vi "GV_DrawLiveBox.vi"(8 "error in (no error)":errorcluster, 11 "Gviewer in":refnum<class "Gviewer.lvclass">) -> (0 "error out":errorcluster, 3 "Gviewer out":refnum<class "Gviewer.lvclass">)   [LabVIEW 2020, in "Gviewer.lvclass"]
doc: "Position Live box on toolbar and update value from attributes"
uses:
  Gviewer.lvclass
  <vilib>/Utility/miscctls.llb/LVPositionTypeDef.ctl
  Gviewer.lvclass/Gviewer.ctl
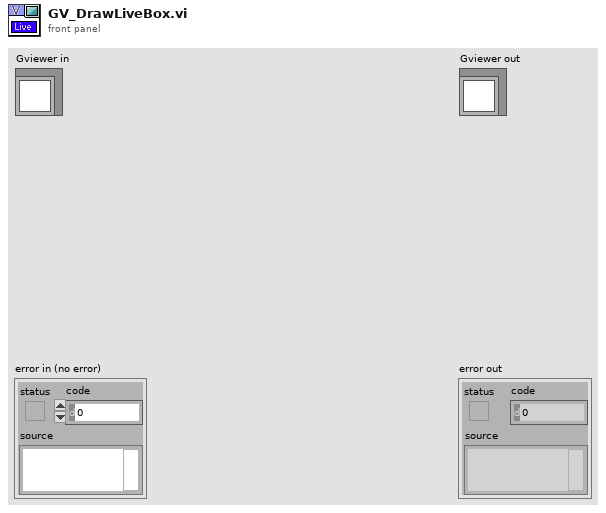
[diagram p1: front panel]
types:
  T1 = typedef "LVPositionTypeDef.ctl" = cluster{"Left":i32, "Top":i32}
  T2 = typedef "Gviewer.lvclass/Typedef_Live.ctl" = enum16{"Live View", "Freeze"}
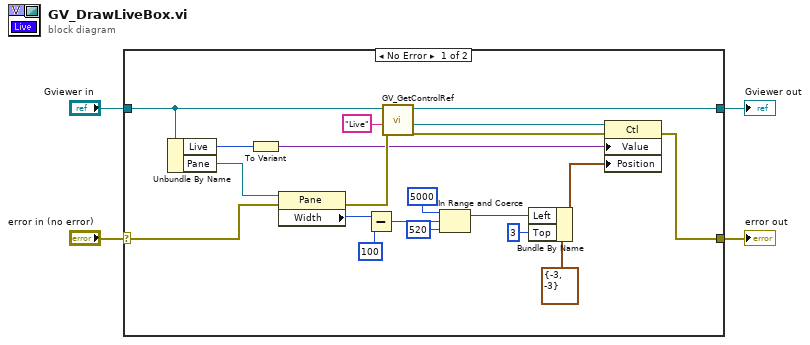
[diagram p0: block diagram]
diagram:
  n1 = case shown="No Error" "error in (no error)" {
    selector: "error in (no error)" -> [w17 w26]
    tunnel: [w16 w26] -> w3
    tunnel: [w18 w25] -> w1
    tunnel: "Gviewer in" -> [w19 w25]
    frame No Error {
      n2 = Unbundle By Name(w19) -> ("Live"=w10:T2, "Pane"=w20:refnum<vi>)
      n3 = To Variant(anything=w10) -> (Variant=w9:variant)
      n4 = property class="Pane"(reference=w20, error in=w17) -> (error out=w21:errorcluster, "Width"=w14:u32)  [unwired: 1 out]
      n5 = Subtract(x=w14, y=u32 100) -> (x-y=w8:u32)
      n6 = call "GV_GetControlRef.vi"("error in (no error)"=w21, "CNT name"="Live", "Gviewer in"=w19) -> ("error out"=w22:errorcluster, "Reference"=w23:refnum<vi>, "Gviewer out"=w18:refnum<class "Gviewer.lvclass">)  [unwired: 6 in]
      n7 = In Range and Coerce(upper limit=u32 5000, x=w8, lower limit=u32 520) -> (coerced(x)=w7:u32)  [unwired: 1 out]
      n8 = Bundle By Name(cluster=T1 {"Left"=-3, "Top"=-3} ("Position"), "Left"=w7, "Top"=3) -> (w11:T1)
      n9 = property class="Ctl"(reference=w23, error in=w22, "Value"=w9, "Position"=w11) -> (error out=w16:errorcluster)  [unwired: 1 out]
    }
    frame Error {
    }
  }
  "error out" <- w3
  "Gviewer out" <- w1
